vi "CODMn测量数据储存.vi"   [LabVIEW 2016, in "斯坦道CODMn新电路板.lvlib"]
types:
  T1 = enum16{"空闲", "水样测试", "标样核查", "零点核查", "跨度核查", "空白测试", "平行样测试", "加标回收", "空白校准", "标样校准", "初始化（清洗）"}
  T2 = enum16{"水样测试", "标样核查", "跨度核查", "零点核查", "空白测试", "加标回收", "空白校准", "标样校准"}
  T3 = cluster{"时间标识":timestamp, "监测值":sgl, "单位":u16, "数据标识":string, "因子编码":u32, "标样参考值":sgl, "A":sgl, "B":sgl, "K":sgl, "终点滴定数":sgl, "环境温度":sgl, "环境湿度":sgl, "量程":sgl, "加热实时温度":sgl}
  T4 = enum16{"维护数据", "水样测试", "标样核查", "零点核查", "跨度核查", "空白测试", "平行样测试", "加标回收", "空白校准", "标样校准", "初始化（清洗）"}
  T5 = cluster{"运行模式":enum16{"维护模式", "常规模式", "应急模式", "质控模式"}, "质控频次":enum16{"关闭", "每天", "星期一", "星期二", "星期三", "星期四", "星期五", "星期六", "星期日"}, "空白核查时间":u16, "跨度核查时间":u16, "24H周期设置":bool[]}
  T6 = cluster{"系统时间":timestamp, "工作状态":u16, "测量模式":enum16{"待机", "连续模式", "周期模式", "定点模式", "受控模式", "手动模式"}, "告警代码":u16, "故障代码":u16, "日志代码":u16, "软件版本":u16, "A":sgl, "B":sgl, "K":sgl, "当前滴定数":sgl, "T":sgl, "H":sgl, "id":u16, "flowid":u16, "量程":u16, "加热实时温度":sgl, "当前ORP值":sgl, "运行时间":sgl, "当前步骤剩余时间":sgl, "结束滴定数":sgl, "注射泵保温温度":sgl}
  T7 = cluster{"因子编码":u32, "单位":u16, "标样参考值":sgl, "水样数据时间":timestamp, "水样实测值":sgl, "水样数据标识":string, "标样数据时间":timestamp, "标样实测值":sgl, "标样数据标识":string, "空白数据时间":timestamp, "空白实测值":sgl, "空白数据标识":string, "零点核查数据时间":timestamp, "零点核查实测值":sgl, "零点核查数据标识":string, "跨度核查数据时间":timestamp, "跨度核查实测值":sgl, "跨度核查数据标识":string, "加标回收数据时间":timestamp, "加标回收实测值":sgl, "加标回收数据标识":string, "平行样数据时间":timestamp, "平行样实测值":sgl, "平行样数据标识":string, "F0":sgl, "F1":sgl, "F2":sgl, "F3":sgl, "F4":sgl, "F5":sgl, "F6":sgl, "F7":sgl, "温度":sgl, "湿度":sgl, "X值":sgl, "fidrange":u16}
  T8 = cluster{"跨度值":dbl, "零点标准液浓度":dbl, "跨度标准液浓度":dbl, "标准液标准浓度":dbl}
  T9 = cluster{"公式":cluster{"X^2":dbl, "X":dbl, "B":dbl}, "校准":cluster{"校准？":bool, "校准点1-5":u16, "校准浓度":dbl}}
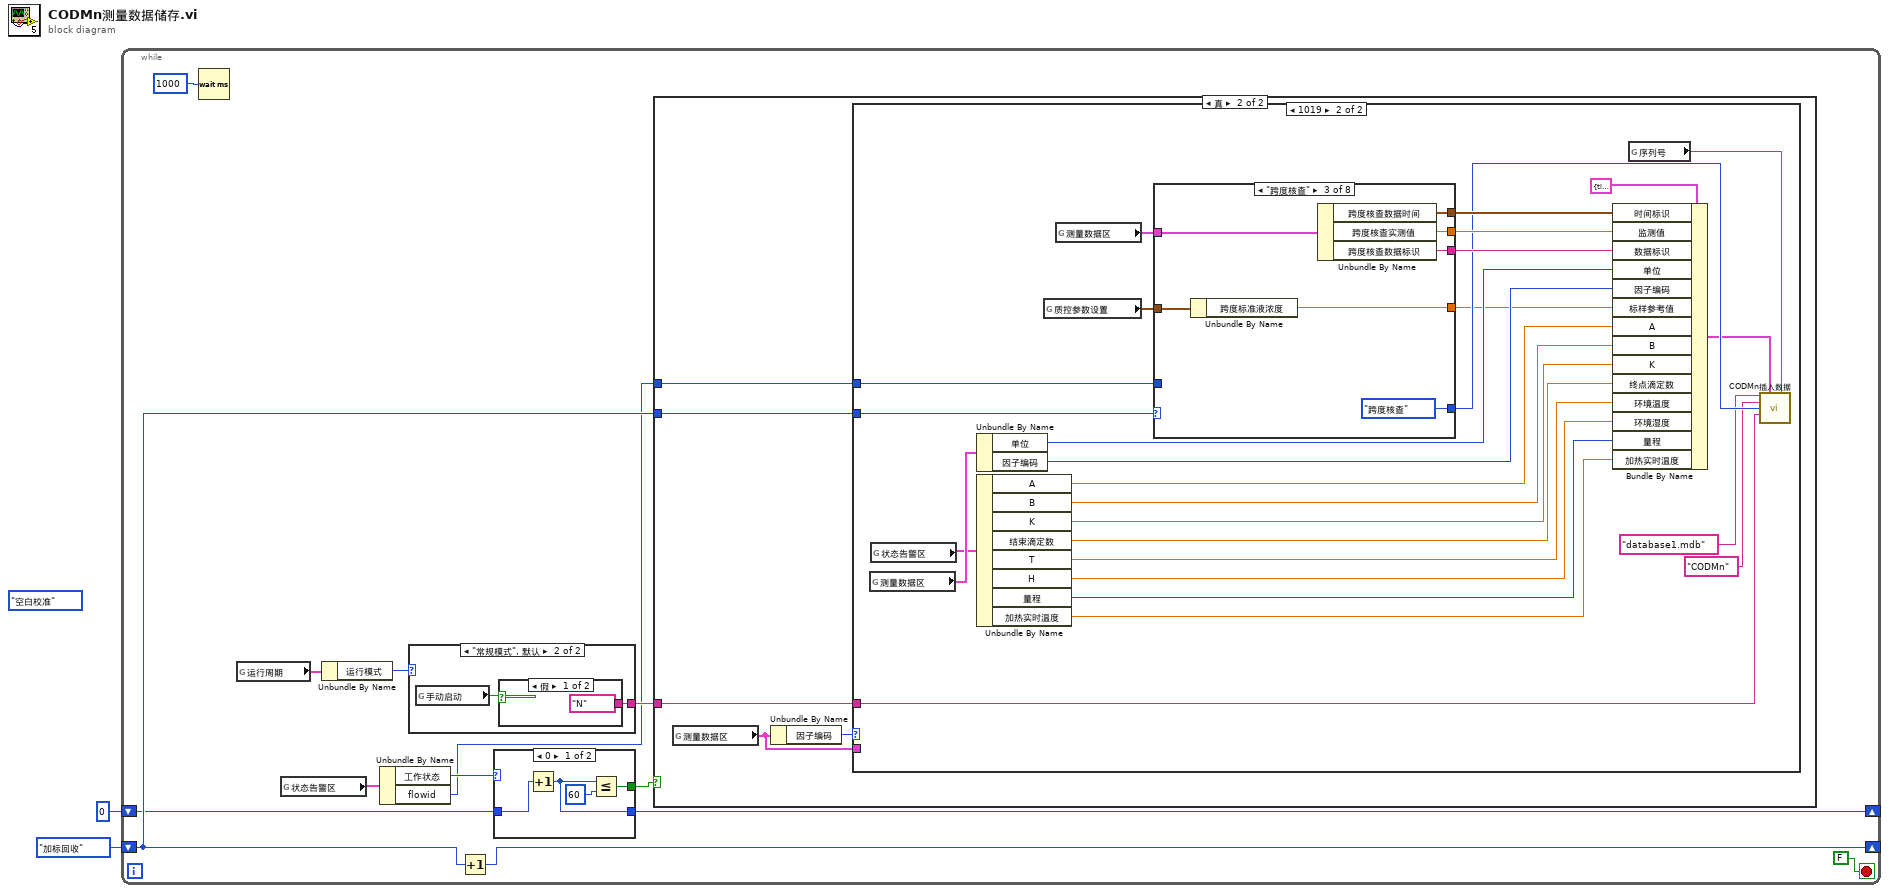
[diagram p0: block diagram]
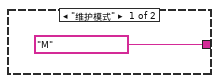
[diagram p2: hidden frame]
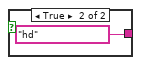
[diagram p3: hidden frame]
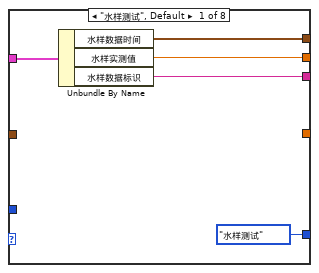
[diagram p7: hidden frame]
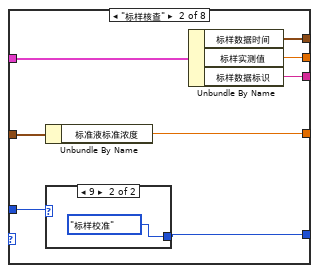
[diagram p8: hidden frame]
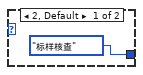
[diagram p9: hidden frame]
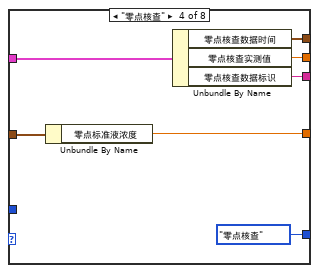
[diagram p10: hidden frame]
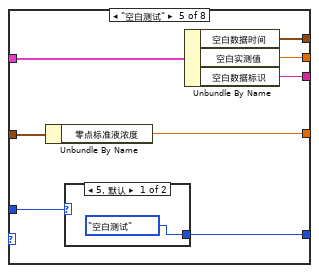
[diagram p11: hidden frame]
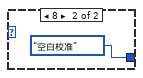
[diagram p12: hidden frame]
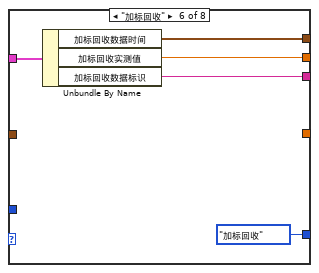
[diagram p13: hidden frame]
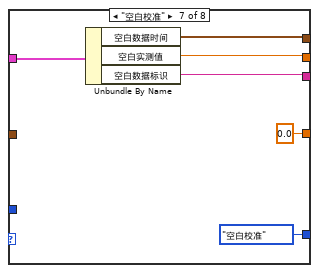
[diagram p14: hidden frame]
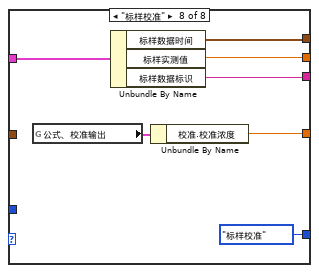
[diagram p15: hidden frame]
diagram:
  (unwired) T1."空白校准" ("工作状态")
  n1 = while {
    shift-right: [w12] -> _
    shift-left: T2."加标回收" ("测量模式") -> [w11]
    shift-right: [w7] -> _
    shift-left: u32 0 ("等待时间（毫秒）") -> [w8]
    stop <- FALSE stop-if-true
    n2 = Wait (ms)(milliseconds to wait=u32 1000 ("等待时间（毫秒）")) -> ()  [unwired: 1 out]
    n3 = global read "CODMn断电保存全局变量.vi" "运行周期"() -> (w4:T5)
    n4 = global read "VARCODMn全局变量.vi" "状态告警区"() -> (w10:T6)
    n5 = Unbundle By Name(w4) -> ("运行模式"=w3:enum16{"维护模式", "常规模式", "应急模式", "质控模式"})
    n6 = Unbundle By Name(w10) -> ("工作状态"=w9:u16, "flowid"=w5:u16)
    n7 = case shown="\"常规模式\", 默认" w3 {
      tunnel: ["M" ("数据标记表") w18] -> w13
      frame "维护模式" {
      }
      frame "常规模式", Default {
        n8 = global read "VARCODMn全局变量.vi" "手动启动"() -> (w17:bool)
        n9 = case shown="假" w17 {
          tunnel: ["N" ("数据标记表") "hd" ("数据标记表")] -> w18
          frame False {
          }
          frame True {
          }
        }
      }
    }
    n10 = Increment(x=w11) -> (x+1=w12:T2)
    n11 = case shown="0" w9 {
      tunnel: w8 -> [w24 _]
      tunnel: [w23 _] -> w7
      tunnel: [w21 _] -> w6
      frame 0 {
        n12 = Increment(x=w24) -> (x+1=w23:u32)
        n13 = Less Or Equal?(x=w23, y=u32 60) -> (x <= y?=w21:bool)
      }
      frame 1, Default {
      }
    }
    n14 = case shown="真" w6 {
      tunnel: w13 -> [_ w27]
      tunnel: w11 -> [_ w26]
      tunnel: w5 -> [_ w25]
      frame False {
      }
      frame True {
        n15 = global read "VARCODMn全局变量.vi" "测量数据区"() -> (w29:T7)
        n16 = Unbundle By Name(w29) -> ("因子编码"=w28:u32)
        n17 = case shown="1019" w28 {
          tunnel: w29 -> [_ _]
          tunnel: w27 -> [_ w45]
          tunnel: w26 -> [_ w44]
          tunnel: w25 -> [_ w41]
          frame Default {
          }
          frame 1019 {
            n18 = global read "VARCODMn全局变量.vi" "测量数据区"() -> (w53:T7)
            n19 = global read "VARCODMn全局变量.vi" "状态告警区"() -> (w40:T6)
            n20 = Unbundle By Name(w53) -> ("单位"=w55:u16, "因子编码"=w54:u32)
            n21 = Unbundle By Name(w40) -> ("A"=w33:sgl, "B"=w39:sgl, "K"=w34:sgl, "结束滴定数"=w35:sgl, "T"=w36:sgl, "H"=w30:sgl, "量程"=w37:u16, "加热实时温度"=w38:sgl)
            n22 = global read "CODMn断电保存全局变量.vi" "质控参数设置"() -> (w43:T8)
            n23 = global read "VARCODMn全局变量.vi" "测量数据区"() -> (w56:T7)
            n24 = case shown="\"跨度核查\"" w44 {
              tunnel: w56 -> [w61 w69 w78 w85 w93 w100 w106 w113]
              tunnel: [w60 w68 w77 w84 w92 w99 w105 w112] -> w49
              tunnel: [w57 w67 w76 w83 w91 w96 w104 w111] -> w50
              tunnel: [w59 w66 w75 w82 w90 w98 w103 w110] -> w51
              tunnel: [T4."水样测试" ("测量模式") w62 T4."跨度核查" ("测量模式") T4."零点核查" ("测量模式") w86 T4."加标回收" ("测量模式") T4."空白校准" ("测量模式") T4."标样校准" ("测量模式")] -> w48
              tunnel: w43 -> [_ w65 w73 w80 w89 _ _ _]
              tunnel: [_ w64 w72 w79 w88 _ 0.0 ("零点标准液浓度") w107] -> w42
              tunnel: w41 -> [_ w63 _ _ w87 _ _ _]
              frame "水样测试", Default {
                n25 = Unbundle By Name(w61) -> ("水样数据时间"=w60:timestamp, "水样实测值"=w57:sgl, "水样数据标识"=w59:string)
              }
              frame "标样核查" {
                n26 = Unbundle By Name(w65) -> ("标准液标准浓度"=w64:dbl)
                n27 = case shown="9" w63 {
                  tunnel: [T4."标样核查" ("测量模式") T4."标样校准" ("测量模式")] -> w62
                  frame 2, Default {
                  }
                  frame 9 {
                  }
                }
                n28 = Unbundle By Name(w69) -> ("标样数据时间"=w68:timestamp, "标样实测值"=w67:sgl, "标样数据标识"=w66:string)
              }
              frame "跨度核查" {
                n29 = Unbundle By Name(w73) -> ("跨度标准液浓度"=w72:dbl)
                n30 = Unbundle By Name(w78) -> ("跨度核查数据时间"=w77:timestamp, "跨度核查实测值"=w76:sgl, "跨度核查数据标识"=w75:string)
              }
              frame "零点核查" {
                n31 = Unbundle By Name(w80) -> ("零点标准液浓度"=w79:dbl)
                n32 = Unbundle By Name(w85) -> ("零点核查数据时间"=w84:timestamp, "零点核查实测值"=w83:sgl, "零点核查数据标识"=w82:string)
              }
              frame "空白测试" {
                n33 = Unbundle By Name(w89) -> ("零点标准液浓度"=w88:dbl)
                n34 = case shown="5, 默认" w87 {
                  tunnel: [T4."空白测试" ("测量模式") T4."空白校准" ("测量模式")] -> w86
                  frame 5, Default {
                  }
                  frame 8 {
                  }
                }
                n35 = Unbundle By Name(w93) -> ("空白数据时间"=w92:timestamp, "空白实测值"=w91:sgl, "空白数据标识"=w90:string)
              }
              frame "加标回收" {
                n36 = Unbundle By Name(w100) -> ("加标回收数据时间"=w99:timestamp, "加标回收实测值"=w96:sgl, "加标回收数据标识"=w98:string)
              }
              frame "空白校准" {
                n37 = Unbundle By Name(w106) -> ("空白数据时间"=w105:timestamp, "空白实测值"=w104:sgl, "空白数据标识"=w103:string)
              }
              frame "标样校准" {
                n38 = global read "CODMn断电保存全局变量.vi" "公式、校准输出"() -> (w108:T9)
                n39 = Unbundle By Name(w113) -> ("标样数据时间"=w112:timestamp, "标样实测值"=w111:sgl, "标样数据标识"=w110:string)
                n40 = Unbundle By Name(w108) -> ("校准.校准浓度"=w107:dbl)
              }
            }
            n41 = Bundle By Name(cluster=T3 {"时间标识"=timestamp(0 s since 1904-01-01), "监测值"=0.0, "单位"=0, "数据标识"="", "因子编码"=0, "标样参考值"=0.0, "A"=0.0, "B"=0.0, "K"=0.0, "终点滴定数"=0.0, "环境温度"=0.0, "环境湿度"=0.0, "量程"=0.0, "加热实时温度"=0.0} ("data"), "时间标识"=w49, "监测值"=w50, "数据标识"=w51, "单位"=w55, "因子编码"=w54, "标样参考值"=w42, "A"=w33, "B"=w39, "K"=w34, "终点滴定数"=w35, "环境温度"=w36, "环境湿度"=w30, "量程"=w37, "加热实时温度"=w38) -> (w31:T3)
            n42 = global read "VARCODMn全局变量.vi" "序列号"() -> (w52:string)
            n43 = call "CODMn插入数据.vi"("database"="database1.mdb", "data"=w31, "SN"=w52, "table"="CODMn", "测量模式"=w48, "数据标记表"=w45) -> ()  [unwired: 9 in, 1 out]
          }
        }
      }
    }
  }
